vi "Use PID.vi"(8 "error in (no error)":errorcluster, 10 "X pixel translation":dbl format="%.2f", 11 "Cascade in":refnum<class "Cascade.lvclass">) -> (0 "error out":errorcluster, 2 "translation out":dbl, 3 "Cascade out":refnum<class "Cascade.lvclass">)   [LabVIEW 2012, in "Cascade.lvclass"]
uses:
  Cascade.lvclass
  Cascade.lvclass/Cascade.ctl
  <vilib>/addons/control/pid/pid.llb/PID (DBL).vi
  <vilib>/addons/control/pid/NI_PID_pid.lvlib
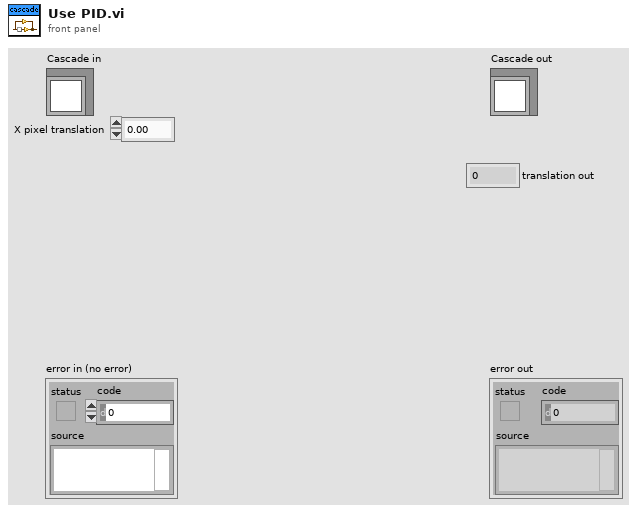
[diagram p1: front panel]
types:
  T1 = cluster{"proportional gain (Kc)":dbl, "integral time (Ti, min)":dbl, "derivative time (Td, min)":dbl}
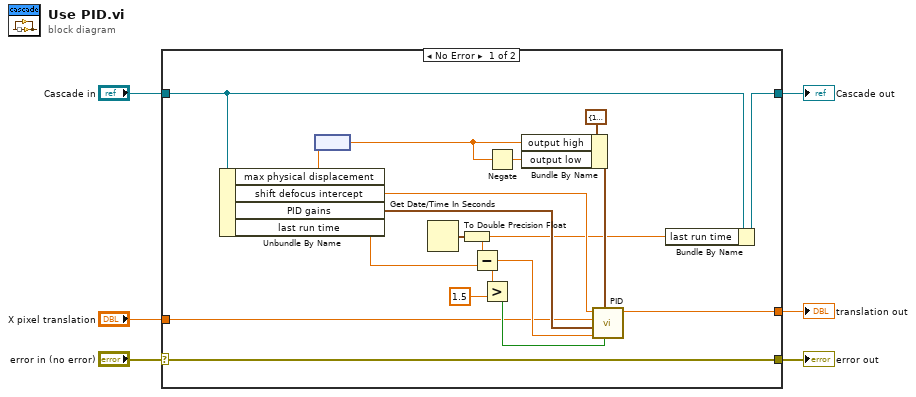
[diagram p0: block diagram]
diagram:
  n1 = case shown="No Error" "error in (no error)" {
    selector: "error in (no error)" -> [w24 w26]
    tunnel: [w24 w26] -> w5
    tunnel: [w10 w25] -> w3
    tunnel: "Cascade in" -> [w11 w25]
    tunnel: "X pixel translation" -> [w8 _]
    tunnel: [w7 _] -> w1
    frame No Error {
      n2 = Unbundle By Name(w11) -> ("max physical displacement"=w12:dbl[unit], "shift defocus intercept"=w13:dbl, "PID gains"=w14:T1, "last run time"=w15:dbl)
      n3 = node(w12) -> (w18:dbl)
      n4 = Get Date/Time In Seconds() -> (seconds since 1Jan1904=w23:timestamp)
      n5 = To Double Precision Float(number=w23) -> (double precision float=w9:dbl)
      n6 = Subtract(x=w9, y=w15) -> (x-y=w17:dbl)
      n7 = Greater?(x=w17, y=1.5) -> (0:w16:bool)
      n8 = Negate(x=w18) -> (-x=w19:dbl)
      n9 = Bundle By Name(cluster=cluster{"output high":dbl, "output low":dbl} {"output high"=100.0, "output low"=-100.0} ("output range"), "output high"=w18, "output low"=w19) -> (w20:cluster{"output high":dbl, "output low":dbl})
      n10 = call-poly <vilib>:"PID.vi"("reinitialize? (F)"=w16, "output range"=w20, "dt (s)"=w17, "PID gains"=w14, "process variable"=w8, "setpoint"=w13) -> ("output"=w7:dbl)  [unwired: 4 in, 1 out]
      n11 = Bundle By Name(cluster=w11, "last run time"=w9) -> (w10:refnum<class "Cascade.lvclass">)
    }
    frame Error {
    }
  }
  "error out" <- w5
  "Cascade out" <- w3
  "translation out" <- w1
